vi "State Machine.vi"() -> ()   [LabVIEW 2017]
uses:
  D:/upwork/Laser Measurement Tool/Laser/tests/KIM101/Thorlabs.MotionControl.KCube.InertialMotorCLI.dll
  Thorlabs.MotionControl.KCube.InertialMotorCLI.dll
  D:/upwork/Laser Measurement Tool/Laser/tests/KIM101/Thorlabs.MotionControl.Controls.dll
  Thorlabs.MotionControl.Controls.dll
panel:
  in  "MoveToReal":bool
  in  "position real":dbl
  in  "Set Feedback Parameters":bool
  in  "FeedbackSignalMode":i32(ring) items=["Disabled", "LimitSwitch", "Encoder"]
  in  "EncoderConst":i32
  in  "Get Feedback Parameters":bool
  out "FeedbackSignalMode":i32(ring) items=["Disabled", "LimitSwitch", "Encoder"]
  out "EncoderConst":i32
  out "Position":i32
  in  "MoveTo":bool
  in  "position":i32
  in  "Jog":bool
  in  "direction":i32(ring)=1 items=["Increase"=1, "Decrease"=2]
  in  "Get Position":bool
  in  "Channel":i32(ring)=1 items=["Channel1"=1, "Channel2"=2, "Channel3"=3, "Channel4"=4]
  out "Position":i32
  in  "Exit":bool
  out "CreateDevice Result":bool
  in  "SerialNumber":string="97000001"
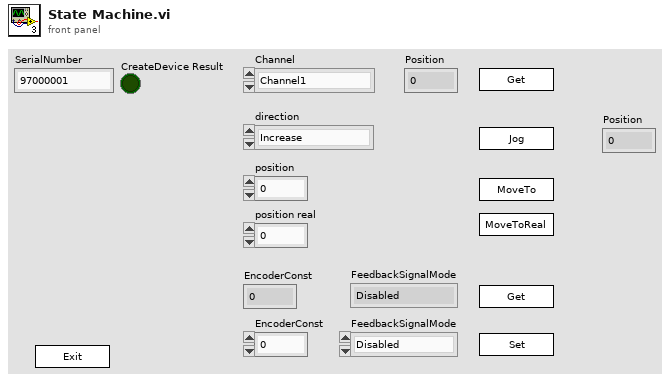
[diagram p1: front panel]
types:
  T1 = enum32{"Invalid", "Standard", "Closed", "Hidden", "Minimized", "Maximized"}
  T2 = enum32{"invalid app kind", "Development System", "Run Time System", "Student Edition", "Embedded LabVIEW", "Evaluation", "Custom"}
  T3 = cluster{"Core":cluster{"Current VI Reference":refnum<vi>, "Close Panel on Exit?":bool}, "KCubeInertialMotorControl":refnum<k24>, "Device":refnum<k24>, "Notifier":refnum<notifier>}
  T4 = cluster{"Current VI Reference":refnum<vi>, "Close Panel on Exit?":bool}
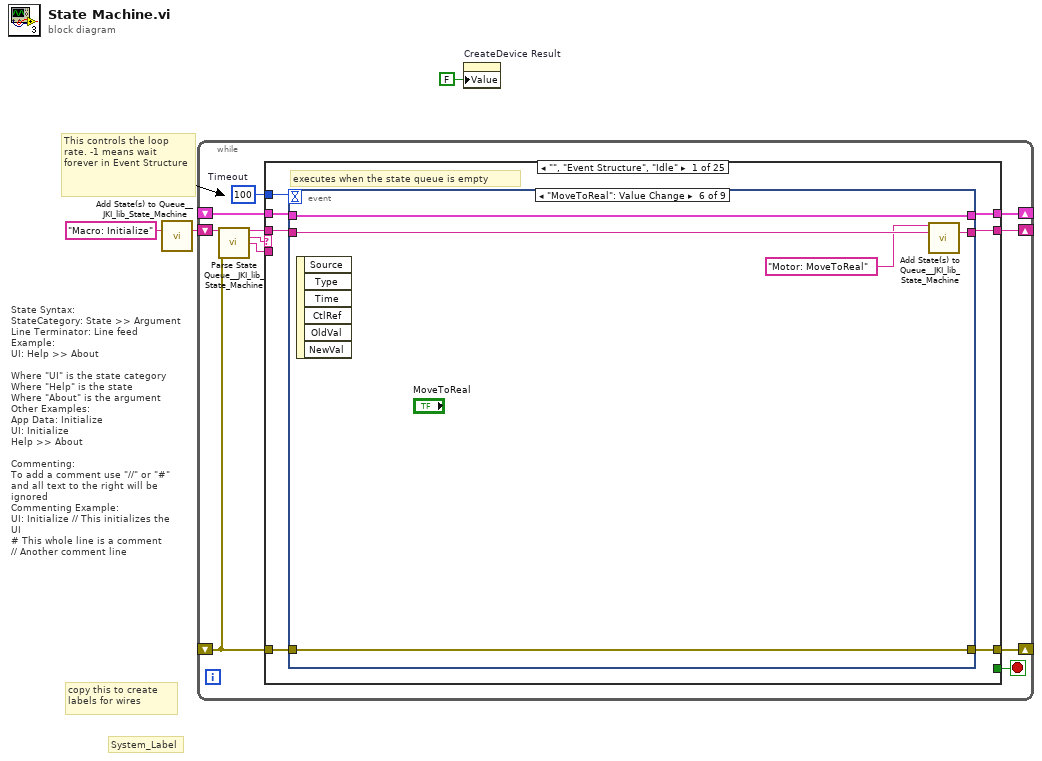
[diagram p0: block diagram]
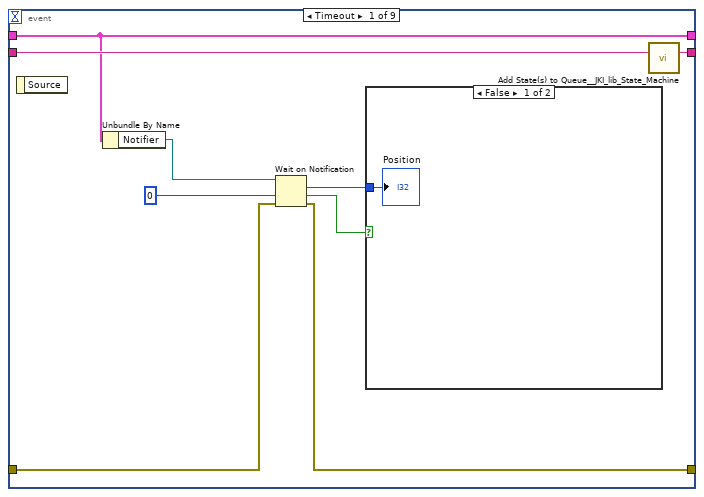
[diagram p2: hidden frame]
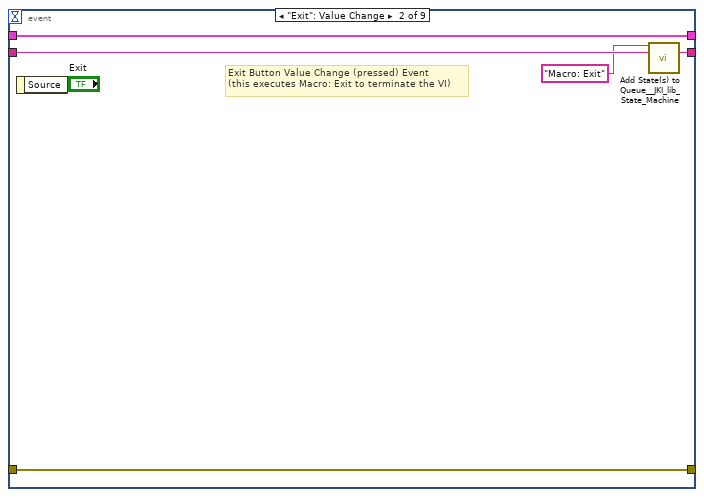
[diagram p4: hidden frame]
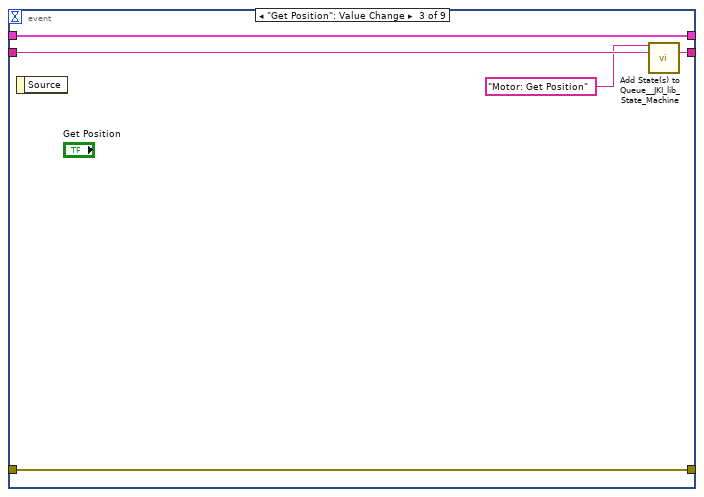
[diagram p5: hidden frame]
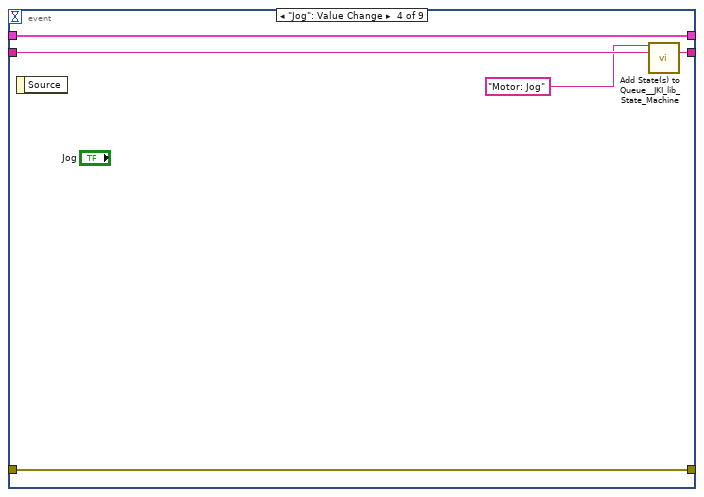
[diagram p6: hidden frame]
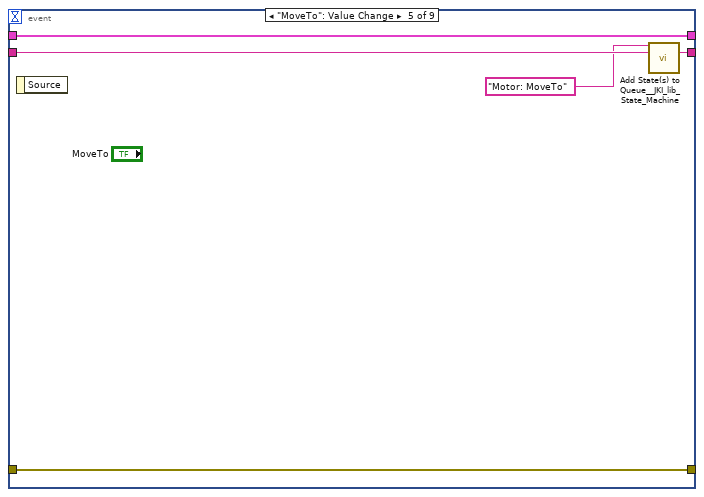
[diagram p7: hidden frame]
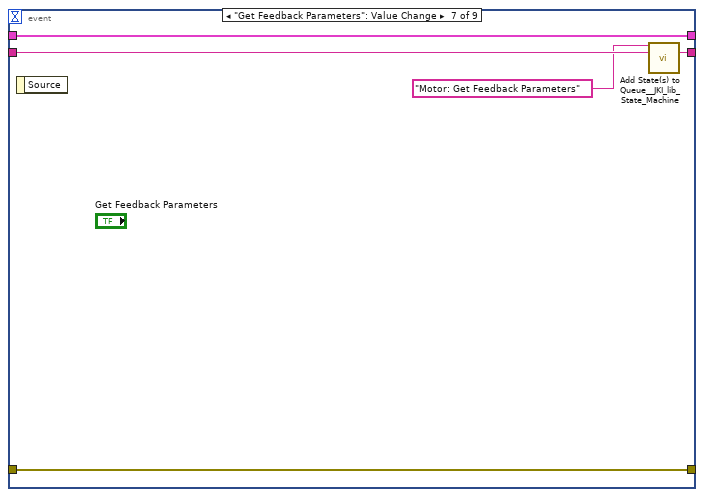
[diagram p8: hidden frame]
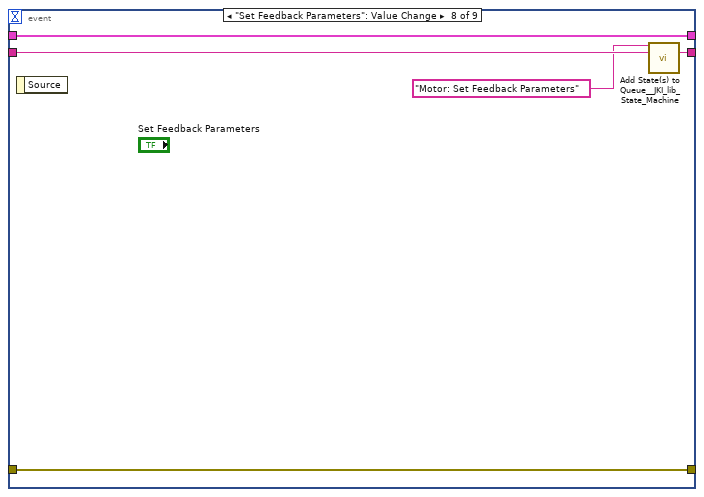
[diagram p9: hidden frame]
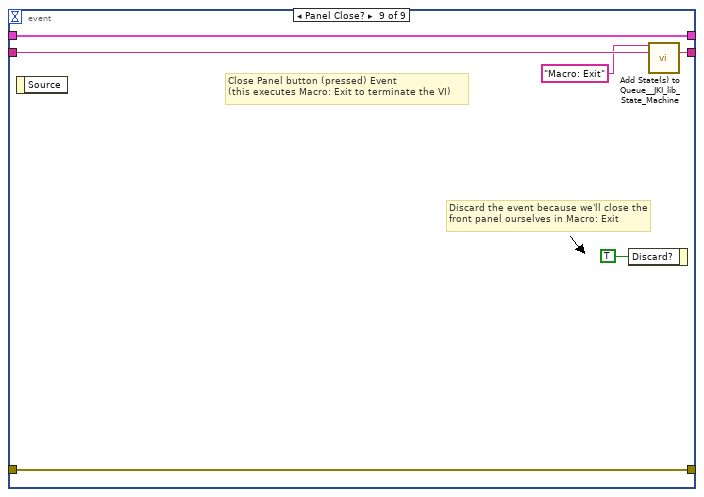
[diagram p10: hidden frame]
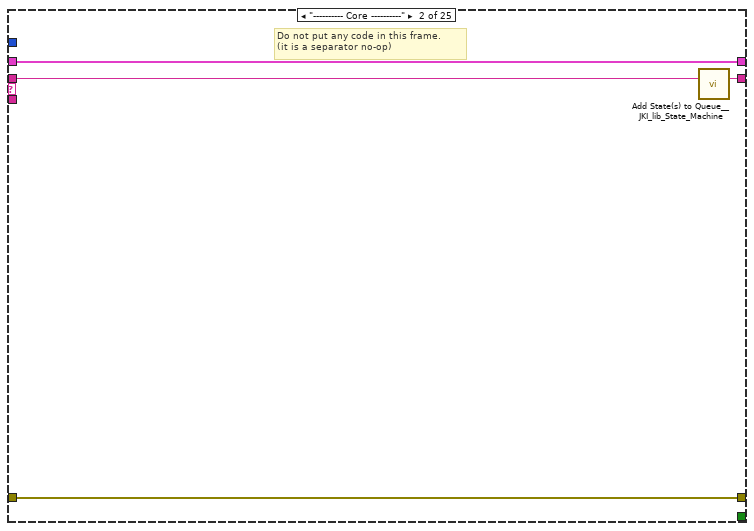
[diagram p11: hidden frame]
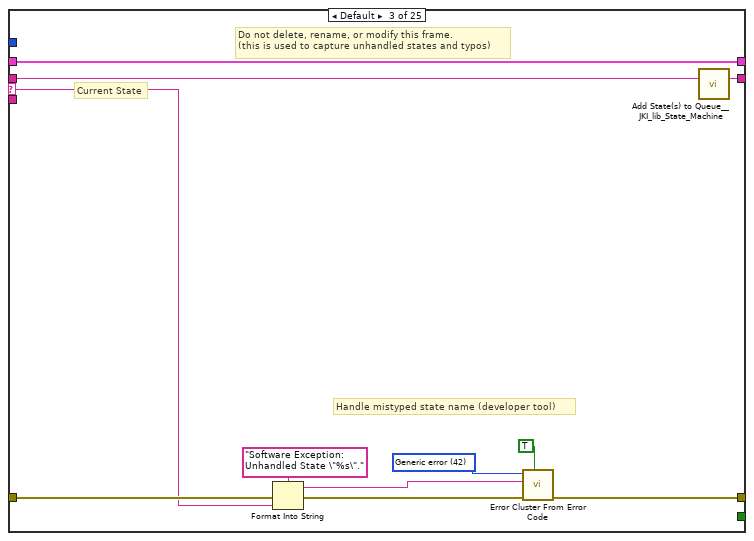
[diagram p12: hidden frame]
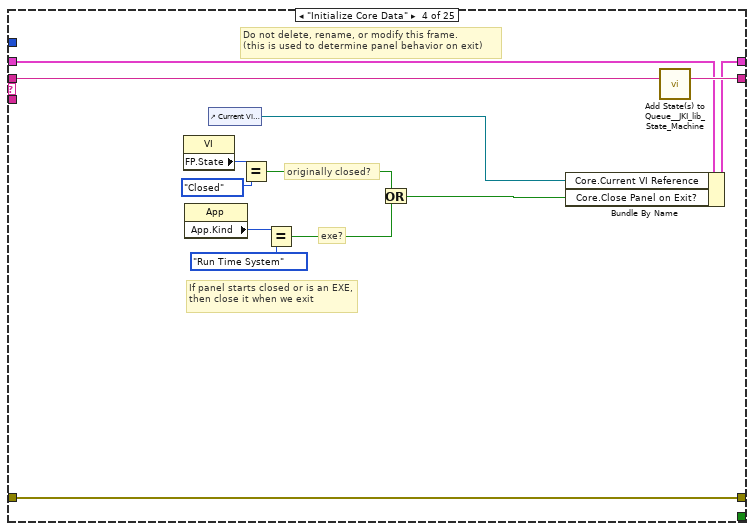
[diagram p13: hidden frame]
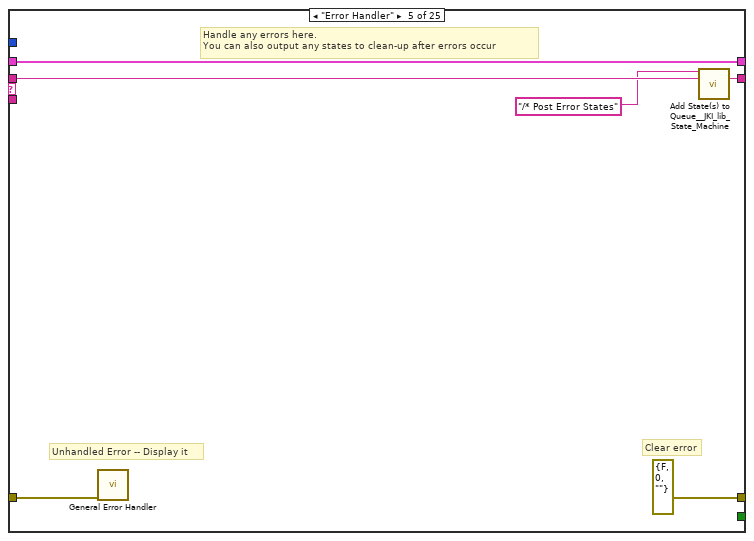
[diagram p14: hidden frame]
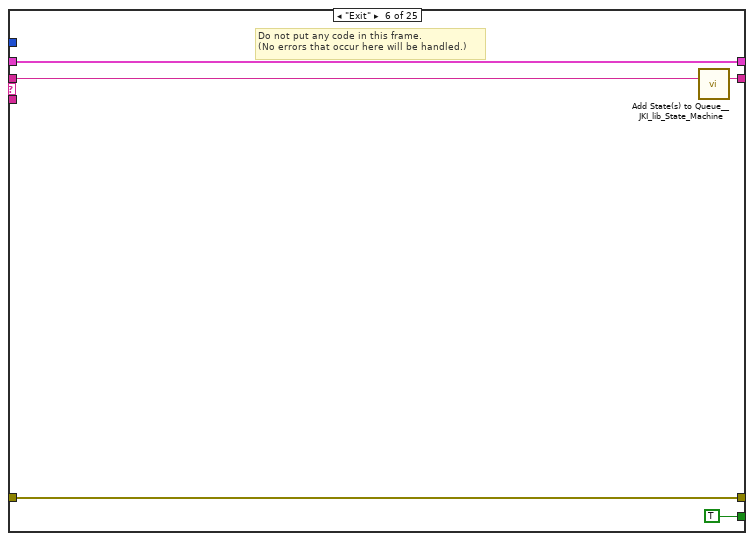
[diagram p15: hidden frame]
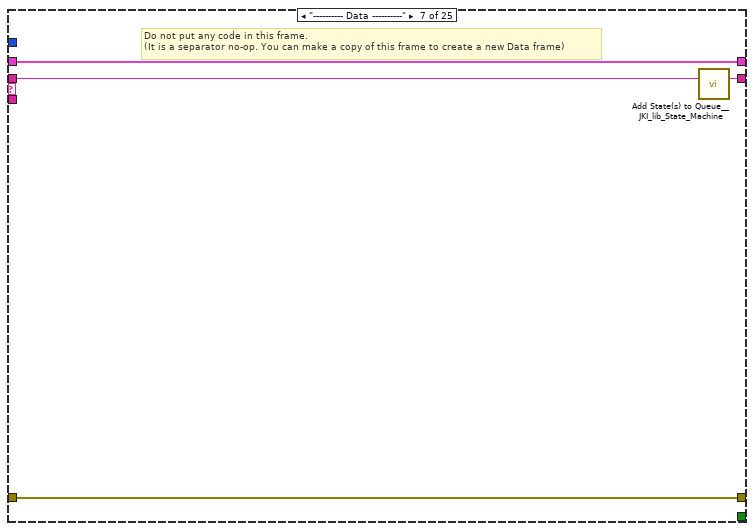
[diagram p16: hidden frame]
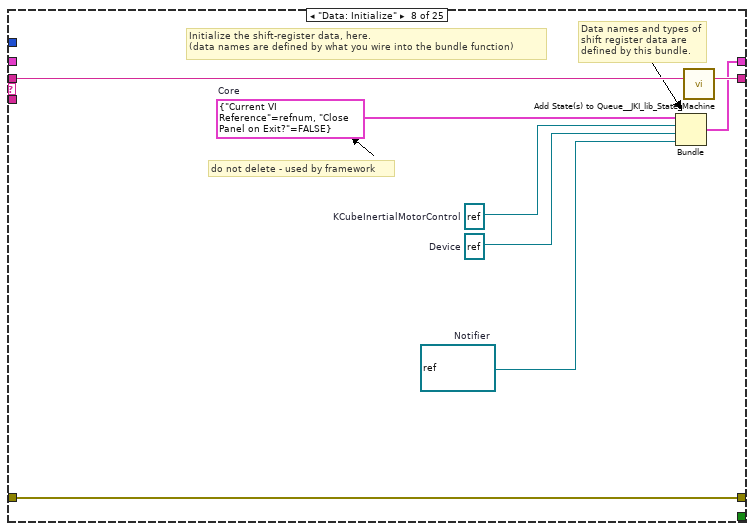
[diagram p17: hidden frame]
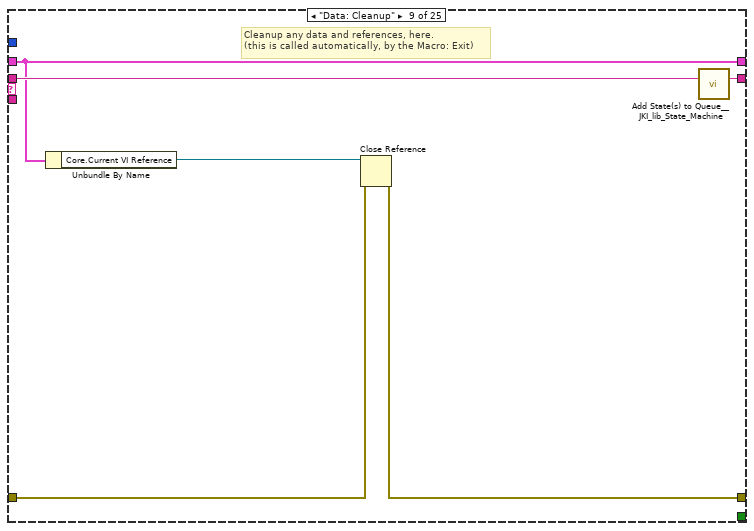
[diagram p18: hidden frame]
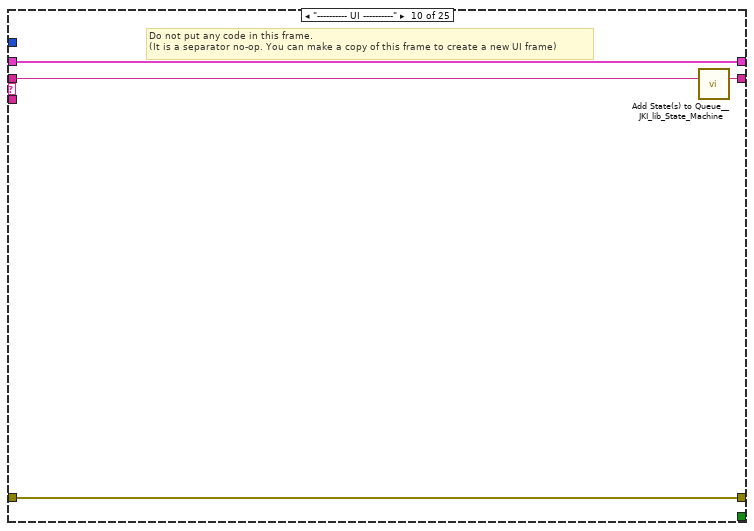
[diagram p19: hidden frame]
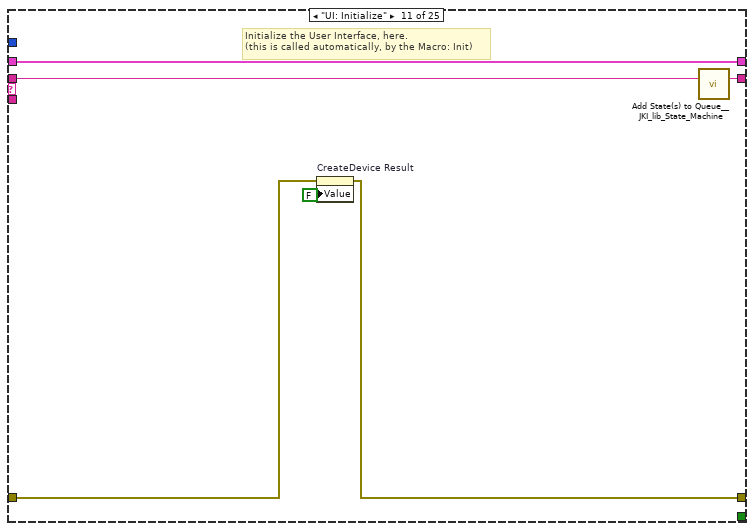
[diagram p20: hidden frame]
diagram:
  # "State Syntax:\nStateCategory: State >> Argument\nLine Terminator: Line feed\nExample:\nUI: Help >> About\n\nWhere \"UI\" is the state category\nWhere \"Help\" is the state\nWhere \"About\" is the argument\nOther Examples:\nApp Data: Initialize\nUI: Initialize\nHelp >> About\n\nCommenting:\nTo add a comment use \"//\" or \"#\" and all text to the right will be ignored\nCommenting Example:\nUI: Initialize // This initializes the UI\n# This whole line is a comment\n// Another comment line"
  # "copy this to create labels for wires"
  # "This controls the loop rate. -1 means wait forever in Event Structure"
  # "System_Label"
  n1 = call <vilib>:"Add State(s) to Queue__JKI_lib_State_Machine.vi"("State(s) in (\"\")"="Macro: Initialize") -> ("States Out"=w3:string)  [unwired: 14 in]
  n2 = while {
    shift-right: [w7] -> _
    shift-left: _ -> [w6]
    shift-right: [w10] -> _
    shift-left: _ -> [w4]
    shift-right: [w9] -> _
    shift-left: w3 -> [w11]
    stop <- w8 stop-if-true
    w5 = 100  # Timeout
    n3 = call <vilib>:"Parse State Queue__JKI_lib_State_Machine.vi"("State Queue"=w11, "Error In (no error)"=w4) -> ("Remaining States"=w13:string, "Current State"=w14:string, "Arguments"=w12:string)  [unwired: 11 in]
    n4 = case shown="\"\", \"Event Structure\", \"Idle\"" w14 {
      selector: w14 -> [_ _ w77 _ _ _ _ _ _ _ _ _ _ _ _ _ _ _ _ _ _ _ _ _ _]
      tunnel: w13 -> [w21 w76 w81 w100 w106 w111 w115 w123 w129 w133 w139 w145 w156 w225 w230 w240 w244 w258 w265 w273 w282 w291 w300 w311 w323]
      tunnel: w12 -> [_ _ _ _ _ _ _ _ _ _ _ w140 w150 _ _ _ _ _ _ _ _ _ _ _ _]
      tunnel: w6 -> [w19 w73 w79 w93 w103 w109 w112 _ w124 w130 w137 w143 w152 w222 w227 w237 w241 w249 w263 w271 w280 w289 w298 w309 w321]
      tunnel: [w18 w74 w83 w97 errorcluster {"status"=FALSE, "code"=0, "source"=""} ("error out") w108 w113 w120 w125 w131 w134 w141 w153 w223 w228 w238 w242 w253 w260 w266 w277 w286 w295 w302 w316] -> w10
      tunnel: w4 -> [w17 w74 w82 w97 w102 w108 w113 w120 w126 w131 w135 w142 w154 w223 w228 w238 w242 w254 w261 w267 w278 w287 w296 w304 _]
      tunnel: [w20 w75 w80 w99 w105 w110 w114 w122 w128 w132 w138 w144 w155 w224 w229 w239 w243 w257 w264 w272 w281 w290 w299 w310 w322] -> w9
      tunnel: [_ _ _ _ _ TRUE _ _ _ _ _ _ _ _ _ _ _ _ _ _ _ _ _ _ _] -> w8
      tunnel: [w16 w73 w79 w98 w103 w109 w112 w121 w124 w130 w137 w143 w152 w222 w227 w237 w241 w251 w263 w271 w280 w289 w298 w309 w321] -> w7
      tunnel: w5 -> [w15 _ _ _ _ _ _ _ _ _ _ _ _ _ _ _ _ _ _ _ _ _ _ _ _]
      frame "", "Event Structure", "Idle" {
        # "executes when the state queue is empty"
        n5 = event shown="[5] \"MoveToReal\": Value Change" {
          selector: _ -> [_ _ _ _ _ _ _ _ _]
          dyn-events: _ -> [_ _ _ _ _ _ _ _ _]
          timeout: w15 -> [_ _ _ _ _ _ _ _ _]
          tunnel: w21 -> [w30 w36 w41 w46 w51 w56 w61 w66 w72]
          tunnel: [w29 w35 w40 w45 w50 w55 w60 w65 w71] -> w20
          tunnel: w19 -> [w28 w33 w38 w43 w48 w53 w58 w63 w69]
          tunnel: [w25 w34 w39 w44 w49 w54 w59 w64 w70] -> w18
          tunnel: w17 -> [w26 w34 w39 w44 w49 w54 w59 w64 w70]
          tunnel: [w28 w33 w38 w43 w48 w53 w58 w63 w69] -> w16
          event Timeout {
            n6 = event-data() -> ()  [unwired: 1 in, 1 out]
            n7 = Unbundle By Name(w28) -> ("Notifier"=w27:refnum<notifier>)
            n8 = Wait on Notification(notifier=w27, timeout in ms (-1)=0, error in (no error)=w26) -> (notification=w22:i32, timed out?=w23:bool, error out=w25:errorcluster)  [unwired: 1 in, 1 out]
            n9 = case shown="False" w23 {
              tunnel: w22 -> [w31 _]
              frame False {
                "Position" <- w31
              }
              frame True {
              }
            }
            n10 = call <vilib>:"Add State(s) to Queue__JKI_lib_State_Machine.vi"("State(s) in (\"\")"=w30) -> ("States Out"=w29:string)  [unwired: 14 in]
          }
          event "Exit": Value Change {
            # "Exit Button Value Change (pressed) Event\n(this executes Macro: Exit to terminate the VI)"
            n11 = event-data() -> ()  [unwired: 1 in, 1 out]
            n12 = call <vilib>:"Add State(s) to Queue__JKI_lib_State_Machine.vi"("State(s) in Front (\"\")"="Macro: Exit", "State(s) in (\"\")"=w36) -> ("States Out"=w35:string)  [unwired: 13 in]
          }
          event "Get Position": Value Change {
            n13 = event-data() -> ()  [unwired: 1 in, 1 out]
            n14 = call <vilib>:"Add State(s) to Queue__JKI_lib_State_Machine.vi"("State(s) in Front (\"\")"="Motor: Get Position", "State(s) in (\"\")"=w41) -> ("States Out"=w40:string)  [unwired: 13 in]
          }
          event "Jog": Value Change {
            n15 = event-data() -> ()  [unwired: 1 in, 1 out]
            n16 = call <vilib>:"Add State(s) to Queue__JKI_lib_State_Machine.vi"("State(s) in Front (\"\")"="Motor: Jog", "State(s) in (\"\")"=w46) -> ("States Out"=w45:string)  [unwired: 13 in]
          }
          event "MoveTo": Value Change {
            n17 = event-data() -> ()  [unwired: 1 in, 1 out]
            n18 = call <vilib>:"Add State(s) to Queue__JKI_lib_State_Machine.vi"("State(s) in Front (\"\")"="Motor: MoveTo", "State(s) in (\"\")"=w51) -> ("States Out"=w50:string)  [unwired: 13 in]
          }
          event "MoveToReal": Value Change {
            n19 = event-data() -> ()  [unwired: 1 in, 6 out]
            n20 = call <vilib>:"Add State(s) to Queue__JKI_lib_State_Machine.vi"("State(s) in Front (\"\")"="Motor: MoveToReal", "State(s) in (\"\")"=w56) -> ("States Out"=w55:string)  [unwired: 13 in]
          }
          event "Get Feedback Parameters": Value Change {
            n21 = event-data() -> ()  [unwired: 1 in, 1 out]
            n22 = call <vilib>:"Add State(s) to Queue__JKI_lib_State_Machine.vi"("State(s) in Front (\"\")"="Motor: Get Feedback Parameters", "State(s) in (\"\")"=w61) -> ("States Out"=w60:string)  [unwired: 13 in]
          }
          event "Set Feedback Parameters": Value Change {
            n23 = event-data() -> ()  [unwired: 1 in, 1 out]
            n24 = call <vilib>:"Add State(s) to Queue__JKI_lib_State_Machine.vi"("State(s) in Front (\"\")"="Motor: Set Feedback Parameters", "State(s) in (\"\")"=w66) -> ("States Out"=w65:string)  [unwired: 13 in]
          }
          event Panel Close? {
            # "Discard the event because we'll close the front panel ourselves in Macro: Exit"
            # "Close Panel button (pressed) Event\n(this executes Macro: Exit to terminate the VI)"
            n25 = event-data() -> ()  [unwired: 1 in, 1 out]
            n26 = event-data("Discard?"=TRUE) -> ()  [unwired: 1 in, 1 out]
            n27 = call <vilib>:"Add State(s) to Queue__JKI_lib_State_Machine.vi"("State(s) in Front (\"\")"="Macro: Exit", "State(s) in (\"\")"=w72) -> ("States Out"=w71:string)  [unwired: 13 in]
          }
        }
      }
      frame "---------- Core ----------" {
        # "Do not put any code in this frame.\n(it is a separator no-op)"
        n28 = call <vilib>:"Add State(s) to Queue__JKI_lib_State_Machine.vi"("State(s) in (\"\")"=w76) -> ("States Out"=w75:string)  [unwired: 14 in]
      }
      frame Default {
        w86 = 42 items=["No error", "Argument error", "Memory is full", "Out of zone", "End of file", "File already open", "Generic file I/O error", "File not found", "File permission error", "Disk is full", "Duplicate path", "Too many files open", "System feature not enabled", "Resource file not found", "Cannot add resource", "Resource not found", "Image not found", "Image memory error", "Pen does not exist", "Config type invalid", "Config token not found", "Config parse error", "Config memory error", "Bad external code format", "Bad external code offset", "External code not present", "Null window", "Destroy window error", "Null menu", "Print aborted", "Bad print record", "Print driver error", "Windows error during printing", "Memory error during printing", "Print dialog error", "Generic print error", "Invalid device refnum", "Device not found", "Device parameter error", "Device unit error", "Cannot open device", "Device call aborted", "Generic error", "Cancelled by user", "Object ID too low", "Object ID too high", "Object not in heap", "Unknown heap", "Unknown object (invalid DefProc)", "Unknown object (DefProc not in table)", "Message out of range", "Invalid (null) method", "Unknown message", "Manager call not supported", "Bad address", "Network operation in progress", "Network operation timed out", "Connection is busy", "Network attribute not supported", "Network error", "Address in use", "System out of memory", "Connection aborted", "Connection refused", "Not connected", "Already connected", "Connection closed", "Initialization error (interapplication manager)", "Bad occurrence", "Wait on unbound occurrence handler", "Occurrence queue overflow", "Datalog type conflict", "Unused", "Unrecognized type (interapplication manager)", "Memory corrupt", "Failed to make temporary DLL", "Old CIN version", "Drag socket not found", "Failed to load drop-object", "Failed to register OLE object", "Failed to release OLE object", "Format specifier type mismatch", "Unknown format specifier", "Too few format specifiers", "Too many format specifiers", "Scan failed", "Newer CIN version", "Error converting to variant", "Runtime menu error", "Password tampered", "Variant attribute not found", "Incompatible variant data type", "Event data is not available", "Event Store is not present", "Occurrence is not found", "Event Queue is not created", "Event info is not available", "Refnum passed is NULL", "Error retrieving Class GUID", "Error retrieving CoClass GUID", "Error retrieving TypeLib GUID.", "Bad built application magic bytes.", "Specific driver is different from the specific driver associated with the Logical Name.", "There is no session opened to the class driver.", "Max Error", "MAX - Error with config objects", "MAX - Error loading configuration", "MAX - Group not supported"]
        # "Current State"
        # "Do not delete, rename, or modify this frame.\n(this is used to capture unhandled states and typos)"
        # "Handle mistyped state name (developer tool)"
        n29 = Format Into String(format string="Software Exception: Unhandled State \"%s\"." ("message"), error in=w82, w77) -> (resulting string=w85:string, error out=w84:errorcluster)  [unwired: 1 in]
        n30 = call <vilib>:"Error Cluster From Error Code.vi"("show call chain? (False)"=TRUE, "error in (no error)"=w84, "error message (\"\")"=w85, "error code (0)"=w86) -> ("error out"=w83:errorcluster)  [unwired: 5 in]
        n31 = call <vilib>:"Add State(s) to Queue__JKI_lib_State_Machine.vi"("State(s) in (\"\")"=w81) -> ("States Out"=w80:string)  [unwired: 14 in]
      }
      frame "Initialize Core Data" {
        # "Do not delete, rename, or modify this frame.\n(this is used to determine panel behavior on exit)"
        # "originally closed?"
        # "exe?"
        # "If panel starts closed or is an EXE, then close it when we exit"
        n32 = property class="VI"() -> ("FP.State"=w90:T1)  [unwired: 2 in, 2 out]
        n33 = property class="App"() -> ("App.Kind"=w96:T2)  [unwired: 2 in, 2 out]
        n34 = control-ref of="Current VI Reference"() -> (w91:refnum<vi>)
        n35 = Equal?(x=w90, y=T1."Closed" ("Front Panel Window:State")) -> (x = y?=w88:bool)
        n36 = Equal?(x=w96, y=T2."Run Time System" ("Application:Kind")) -> (x = y?=w94:bool)
        n37 = Or(x=w88, y=w94) -> (x .or. y?=w92:bool)
        n38 = Bundle By Name(cluster=w93, "Core.Current VI Reference"=w91, "Core.Close Panel on Exit?"=w92) -> (w98:T3)
        n39 = call <vilib>:"Add State(s) to Queue__JKI_lib_State_Machine.vi"("State(s) in (\"\")"=w100) -> ("States Out"=w99:string)  [unwired: 14 in]
      }
      frame "Error Handler" {
        # "Unhandled Error -- Display it"
        # "Handle any errors here.\nYou can also output any states to clean-up after errors occur"
        # "Clear error"
        n40 = call <vilib>:"General Error Handler.vi"("error in (no error)"=w102) -> ()  [unwired: 10 in, 5 out]
        n41 = call <vilib>:"Add State(s) to Queue__JKI_lib_State_Machine.vi"("State(s) in Front (\"\")"="/* Post Error States", "State(s) in (\"\")"=w106) -> ("States Out"=w105:string)  [unwired: 13 in]
      }
      frame "Exit" {
        # "Do not put any code in this frame.\n(No errors that occur here will be handled.)"
        n42 = call <vilib>:"Add State(s) to Queue__JKI_lib_State_Machine.vi"("State(s) in (\"\")"=w111) -> ("States Out"=w110:string)  [unwired: 14 in]
      }
      frame "---------- Data ----------" {
        # "Do not put any code in this frame.\n(It is a separator no-op. You can make a copy of this frame to create a new Data frame)"
        n43 = call <vilib>:"Add State(s) to Queue__JKI_lib_State_Machine.vi"("State(s) in (\"\")"=w115) -> ("States Out"=w114:string)  [unwired: 14 in]
      }
      frame "Data: Initialize" {
        w116 = refnum<notifier> refnum  # Notifier
        w117 = refnum<k24> refnum  # Device
        w118 = refnum<k24> refnum  # KCubeInertialMotorControl
        w119 = T4 {"Current VI Reference"=refnum, "Close Panel on Exit?"=FALSE}  # Core
        # "do not delete - used by framework"
        # "Data names and types of shift register data are defined by this bundle."
        # "Initialize the shift-register data, here.\n(data names are defined by what you wire into the bundle function)"
        n44 = Bundle("Core"=w119, "KCubeInertialMotorControl"=w118, "Device"=w117, "Notifier"=w116) -> (w121:T3)  [unwired: 1 in]
        n45 = call <vilib>:"Add State(s) to Queue__JKI_lib_State_Machine.vi"("State(s) in (\"\")"=w123) -> ("States Out"=w122:string)  [unwired: 14 in]
      }
      frame "Data: Cleanup" {
        # "Cleanup any data and references, here.\n(this is called automatically, by the Macro: Exit)"
        n46 = Unbundle By Name(w124) -> ("Core.Current VI Reference"=w127:refnum<vi>)
        n47 = Close Reference(reference=w127, error in (no error)=w126) -> (error out=w125:errorcluster)
        n48 = call <vilib>:"Add State(s) to Queue__JKI_lib_State_Machine.vi"("State(s) in (\"\")"=w129) -> ("States Out"=w128:string)  [unwired: 14 in]
      }
      frame "---------- UI ----------" {
        # "Do not put any code in this frame.\n(It is a separator no-op. You can make a copy of this frame to create a new UI frame)"
        n49 = call <vilib>:"Add State(s) to Queue__JKI_lib_State_Machine.vi"("State(s) in (\"\")"=w133) -> ("States Out"=w132:string)  [unwired: 14 in]
      }
      frame "UI: Initialize" {
        # "Initialize the User Interface, here.\n(this is called automatically, by the Macro: Init)"
        n50 = property on="CreateDevice Result" class="Bool (strict)"(error in=w135, "Value"=FALSE ("CreateDevice Result")) -> (error out=w134:errorcluster)  [unwired: 1 in, 1 out]
        n51 = call <vilib>:"Add State(s) to Queue__JKI_lib_State_Machine.vi"("State(s) in (\"\")"=w139) -> ("States Out"=w138:string)  [unwired: 14 in]
      }
      frame "UI: Cursor Set" {
        # "Argument"
        # "Set and Unset Cursor Busy.\n(Usage: \"UI: Cursor Set >> Busy|Idle\")"
        n52 = case shown="\"Idle\", Default" w140 {
          tunnel: w142 -> [w147 w149]
          tunnel: [w146 w148] -> w141
          frame "Idle", Default {
            n53 = call <vilib>:"Unset Busy.vi"("error in (no error)"=w147) -> ("error out"=w146:errorcluster)  [unwired: 10 in]
          }
          frame "Busy" {
            n54 = call <vilib>:"Set Busy.vi"("error in (no error)"=w149) -> ("error out"=w148:errorcluster)  [unwired: 9 in, 1 out]
          }
        }
        n55 = call <vilib>:"Add State(s) to Queue__JKI_lib_State_Machine.vi"("State(s) in (\"\")"=w145) -> ("States Out"=w144:string)  [unwired: 14 in]
      }
      frame "UI: Front Panel State" {
        # "Argument"
        # "Set Front Panel Open or Closed\n(Usage: \"UI: Front Panel State >> Open|Close\")"
        n56 = Unbundle By Name(w152) -> ("Core.Current VI Reference"=w151:refnum<vi>)
        n57 = case shown="\"Hidden\", \"Hide\"" w150 {
          tunnel: w154 -> [w162 w177 w188 w201 w214]
          tunnel: [w164 w178 w190 w203 w216] -> w153
          tunnel: w151 -> [w163 w175 w189 w202 w215]
          frame "Open", "Standard", Default {
            w157 = T1."Standard" ("State")
            n58 = property class="VI"(reference=w163, error in=w162) -> (reference out=w160:refnum<vi>, error out=w161:errorcluster, "FP.State"=w159:T1)
            n59 = Not Equal?(x=w159, y=w157) -> (x != y?=w158:bool)
            n60 = case shown="True" w158 {
              tunnel: [w168 w170] -> w164
              tunnel: w161 -> [w167 w170]
              tunnel: w160 -> [w166 _]
              tunnel: w157 -> [w165 _]
              frame True {
                n61 = invoke class="VI" method="FP.Open"(reference=w166, error in=w167, "Activate"=TRUE, "State"=w165) -> (error out=w168:errorcluster)  [unwired: 1 in, 4 out]
              }
              frame False {
              }
            }
          }
          frame "Close", "Closed" {
            n62 = property class="VI"(reference=w175, error in=w177) -> (reference out=w174:refnum<vi>, error out=w176:errorcluster, "FP.State"=w172:T1)
            n63 = Not Equal?(x=w172, y=T1."Closed" ("Front Panel Window:State")) -> (x != y?=w171:bool)
            n64 = case shown="True" w171 {
              tunnel: [w179 w182] -> w178
              tunnel: w176 -> [w179 w181]
              tunnel: w174 -> [_ w180]
              frame False {
              }
              frame True {
                n65 = invoke class="VI" method="FP.Close"(reference=w180, error in=w181) -> (error out=w182:errorcluster)  [unwired: 1 in, 2 out]
              }
            }
          }
          frame "Hidden", "Hide" {
            w183 = T1."Hidden" ("State")
            n66 = property class="VI"(reference=w189, error in=w188) -> (reference out=w186:refnum<vi>, error out=w187:errorcluster, "FP.State"=w185:T1)
            n67 = Not Equal?(x=w185, y=w183) -> (x != y?=w184:bool)
            n68 = case shown="True" w184 {
              tunnel: [w194 w195] -> w190
              tunnel: w187 -> [w193 w195]
              tunnel: w186 -> [w192 _]
              tunnel: w183 -> [w191 _]
              frame True {
                n69 = invoke class="VI" method="FP.Open"(reference=w192, error in=w193, "State"=w191) -> (error out=w194:errorcluster)  [unwired: 2 in, 4 out]
              }
              frame False {
              }
            }
          }
          frame "Minimize", "Minimized" {
            w196 = T1."Minimized" ("State")
            n70 = property class="VI"(reference=w202, error in=w201) -> (reference out=w199:refnum<vi>, error out=w200:errorcluster, "FP.State"=w198:T1)
            n71 = Not Equal?(x=w198, y=w196) -> (x != y?=w197:bool)
            n72 = case shown="True" w197 {
              tunnel: [w207 w208] -> w203
              tunnel: w200 -> [w206 w208]
              tunnel: w199 -> [w205 _]
              tunnel: w196 -> [w204 _]
              frame True {
                n73 = invoke class="VI" method="FP.Open"(reference=w205, error in=w206, "State"=w204) -> (error out=w207:errorcluster)  [unwired: 2 in, 4 out]
              }
              frame False {
              }
            }
          }
          frame "Maximize", "Maximized" {
            w209 = T1."Maximized" ("State")
            n74 = property class="VI"(reference=w215, error in=w214) -> (reference out=w212:refnum<vi>, error out=w213:errorcluster, "FP.State"=w211:T1)
            n75 = Not Equal?(x=w211, y=w209) -> (x != y?=w210:bool)
            n76 = case shown="True" w210 {
              tunnel: [w220 w221] -> w216
              tunnel: w213 -> [w219 w221]
              tunnel: w212 -> [w218 _]
              tunnel: w209 -> [w217 _]
              frame True {
                n77 = invoke class="VI" method="FP.Open"(reference=w218, error in=w219, "State"=w217) -> (error out=w220:errorcluster)  [unwired: 2 in, 4 out]
              }
              frame False {
              }
            }
          }
        }
        n78 = call <vilib>:"Add State(s) to Queue__JKI_lib_State_Machine.vi"("State(s) in (\"\")"=w156) -> ("States Out"=w155:string)  [unwired: 14 in]
      }
      frame "---------- Macro ----------" {
        # "Do not put any code in this frame.\n(It is a separator no-op. You can make a copy of this frame to create a new Macro frame)"
        n79 = call <vilib>:"Add State(s) to Queue__JKI_lib_State_Machine.vi"("State(s) in (\"\")"=w225) -> ("States Out"=w224:string)  [unwired: 14 in]
      }
      frame "Macro: Initialize" {
        w226 = "Data: Initialize\nInitialize Core Data\nUI: Initialize\nUI: Front Panel State >> Open\nMotor: Init"  # Data: Initialize Initialize Core Data UI: Initialize UI: Front Panel State >> Open Motor: Init
        # "Initialization Macro\n(This is called once, when the VI starts)"
        n80 = call <vilib>:"Add State(s) to Queue__JKI_lib_State_Machine.vi"("State(s) in Front (\"\")"=w226, "State(s) in (\"\")"=w230) -> ("States Out"=w229:string)  [unwired: 13 in]
      }
      frame "Macro: Exit" {
        # "Exit Macro\n(This is called once, when the VI exits)"
        n81 = Unbundle By Name(w237) -> ("Core.Close Panel on Exit?"=w236:bool)
        n82 = Select(t="UI: Front Panel State >> Close", s=w236, f="") -> (s? t:f=w233:string)
        n83 = call <vilib>:"Add State(s) to Queue__JKI_lib_State_Machine.vi"("State(s) in (\"\")"=w233, "State(s) at Back (\"\")"="Motor: Deinit\nData: Cleanup\nExit") -> ("States Out"=w231:string)  [unwired: 13 in]
        n84 = call <vilib>:"Add State(s) to Queue__JKI_lib_State_Machine.vi"("State(s) in Front (\"\")"=w231, "State(s) in (\"\")"=w240) -> ("States Out"=w239:string)  [unwired: 13 in]
      }
      frame "---------- Motor ----------" {
        # "Template Separator\n(You can make a copy of, or modify, this frame)"
        n85 = call <vilib>:"Add State(s) to Queue__JKI_lib_State_Machine.vi"("State(s) in (\"\")"=w244) -> ("States Out"=w243:string)  [unwired: 14 in]
      }
      frame "Motor: Init" {
        n86 = call "Create Device Reference.vi"("error in (no error)"=w254, "SerialNumber"="SerialNumber") -> ("error out"=w253:errorcluster, "Device"=w245:refnum<k24>, "KCubeInertialMotorControl out"=w252:refnum<k24>, "CreateDevice Result"=→"CreateDevice Result":bool)  [unwired: 6 in]
        n87 = vi-ref "CallBack.vi"() -> ("vi reference"=w250:refnum<vi>)
        n88 = Obtain Notifier(notification data type=0) -> (notifier out=w246:refnum<notifier>)  [unwired: 3 in, 2 out]
        n89 = To Variant(anything=w246) -> (Variant=w248:variant)
        n90 = node(w245, w250, w248) -> ()  [unwired: 2 in, 2 out]
        n91 = Bundle By Name(cluster=w249, "KCubeInertialMotorControl"=w252, "Device"=w245, "Notifier"=w246) -> (w251:T3)
        n92 = call <vilib>:"Add State(s) to Queue__JKI_lib_State_Machine.vi"("State(s) in (\"\")"=w258) -> ("States Out"=w257:string)  [unwired: 14 in]
      }
      frame "Motor: Deinit" {
        n93 = Unbundle By Name(w263) -> ("KCubeInertialMotorControl"=w262:refnum<k24>, "Device"=w259:refnum<k24>)
        n94 = call "Close Device Reference.vi"("error in (no error)"=w261, "Device"=w259, "KCubeInertialMotorControl in"=w262) -> ("error out"=w260:errorcluster)  [unwired: 8 in]
        n95 = call <vilib>:"Add State(s) to Queue__JKI_lib_State_Machine.vi"("State(s) in (\"\")"=w265) -> ("States Out"=w264:string)  [unwired: 14 in]
      }
      frame "Motor: Get Position" {
        n96 = Unbundle By Name(w271) -> ("Device"=w268:refnum<k24>)
        n97 = invoke class="KCubeInertialMotor" method="GetPosition"(reference=w268, error in=w267, "channel"="Channel") -> (error out=w266:errorcluster, "GetPosition"=→"Position":i32)  [unwired: 1 in, 2 out]
        n98 = call <vilib>:"Add State(s) to Queue__JKI_lib_State_Machine.vi"("State(s) in (\"\")"=w273) -> ("States Out"=w272:string)  [unwired: 14 in]
      }
      frame "Motor: Jog" {
        n99 = Unbundle By Name(w280) -> ("Device"=w279:refnum<k24>)
        n100 = property on="Channel" class="Ring (strict)"() -> ("Value"=w276:i32)  [unwired: 2 in, 2 out]
        n101 = invoke class="KCubeInertialMotor" method="Jog"(reference=w279, error in=w278, "channel"=w276, "direction"="direction", "waitTimeout"=10000) -> (error out=w277:errorcluster)  [unwired: 1 in, 5 out]
        n102 = call <vilib>:"Add State(s) to Queue__JKI_lib_State_Machine.vi"("State(s) in (\"\")"=w282) -> ("States Out"=w281:string)  [unwired: 14 in]
      }
      frame "Motor: MoveTo" {
        n103 = Unbundle By Name(w289) -> ("Device"=w288:refnum<k24>)
        n104 = property on="Channel" class="Ring (strict)"() -> ("Value"=w285:i32)  [unwired: 2 in, 2 out]
        n105 = invoke class="KCubeInertialMotor" method="MoveTo"(reference=w288, error in=w287, "channel"=w285, "position"="position", "waitTimeout"=10000) -> (error out=w286:errorcluster)  [unwired: 1 in, 5 out]
        n106 = call <vilib>:"Add State(s) to Queue__JKI_lib_State_Machine.vi"("State(s) in (\"\")"=w291) -> ("States Out"=w290:string)  [unwired: 14 in]
      }
      frame "Motor: MoveToReal" {
        n107 = Unbundle By Name(w298) -> ("Device"=w297:refnum<k24>)
        n108 = property on="Channel" class="Ring (strict)"() -> ("Value"=w294:i32)  [unwired: 2 in, 2 out]
        n109 = invoke class="KCubeInertialMotor" method="MoveTo"(reference=w297, error in=w296, "channel"=w294, "position"="position real", "waitTimeout"=10000) -> (error out=w295:errorcluster)  [unwired: 1 in, 5 out]
        n110 = call <vilib>:"Add State(s) to Queue__JKI_lib_State_Machine.vi"("State(s) in (\"\")"=w300) -> ("States Out"=w299:string)  [unwired: 14 in]
      }
      frame "Motor: Get Feedback Parameters" {
        n111 = property on="Channel" class="Ring (strict)"() -> ("Value"=w307:i32)  [unwired: 2 in, 2 out]
        n112 = Unbundle By Name(w309) -> ("Device"=w308:refnum<k24>)
        n113 = invoke class="KCubeInertialMotor" method="GetFeedbackSigParameters"(reference=w308, error in=w304, "channel"=w307) -> (error out=w303:errorcluster, "GetFeedbackSigParameters"=w301:refnum<k24>)  [unwired: 1 in, 2 out]
        n114 = property class="FeedbackSignalParams"(reference=w301, error in=w303) -> (error out=w302:errorcluster, "EncoderConst"=→"EncoderConst":i32, "FeedbackSignalMode"=→"FeedbackSignalMode":i32)  [unwired: 1 out]
        n115 = call <vilib>:"Add State(s) to Queue__JKI_lib_State_Machine.vi"("State(s) in (\"\")"=w311) -> ("States Out"=w310:string)  [unwired: 14 in]
      }
      frame "Motor: Set Feedback Parameters" {
        n116 = Unbundle By Name(w321) -> ("Device"=w315:refnum<k24>)
        n117 = property on="Channel" class="Ring (strict)"() -> ("Value"=w313:i32)  [unwired: 2 in, 2 out]
        n118 = invoke class="KCubeInertialMotor" method="GetFeedbackSigParameters"(reference=w315, "channel"=w313) -> (reference out=w314:refnum<k24>, "GetFeedbackSigParameters"=w312:refnum<k24>)  [unwired: 2 in, 2 out]
        n119 = property class="FeedbackSignalParams"(reference=w312, "EncoderConst"="EncoderConst", "FeedbackSignalMode"="FeedbackSignalMode") -> (reference out=w320:refnum<k24>, error out=w317:errorcluster)  [unwired: 1 in]
        n120 = invoke class="KCubeInertialMotor" method="SetFeedbackSigParameters"(reference=w314, error in=w317, "channel"=w313, "feedbackSignalParameters"=w320) -> (error out=w316:errorcluster)  [unwired: 1 in, 4 out]
        n121 = call <vilib>:"Add State(s) to Queue__JKI_lib_State_Machine.vi"("State(s) in (\"\")"=w323) -> ("States Out"=w322:string)  [unwired: 14 in]
      }
    }
  }
  n122 = property on="CreateDevice Result" class="Bool (strict)"("Value"=FALSE ("CreateDevice Result")) -> ()  [unwired: 2 in, 2 out]
